vi "DefaultFromIni.vi"(8 "error in (no error)":errorcluster, 11 "CorrFactor in":refnum<class "CorrFactor.lvclass">) -> (0 "error out":errorcluster, 3 "CorrFactor out":refnum<class "CorrFactor.lvclass">)   [LabVIEW 2018, in "AnalysisPlugins.lvlib" / "CorrFactor.lvclass"]
uses:
  CorrFactor.lvclass
  F:/Program Files (x86)/National Instruments/LabVIEW 2018/user.lib/NIST/BaseClasses/BasePlugin_class/BasePlugin.lvclass
  Typedefs/clAnalysisConfig.ctl
  Typedefs/3458 Params.ctl
  <userlib>/NIST/BaseClasses/BasePlugin_class/BasePlugin.lvclass/BasePlugin.ctl
  FGen/MemberClasses/FunctionBaseClass/FunctionBase.lvclass
  CorrFactor.lvclass/CorrFactor.ctl
  <userlib>/NIST/BaseClasses/BasePlugin_class/Accessors/Read PluginIniFilePath.vi
  Accessors/Write 3458_Config.vi
  Accessors/Write FunctionIniFilePath.vi
  Accessors/Write PhaseRange.vi
  Accessors/Write Function.vi
  <vilib>/Utility/error.llb/Error Cluster From Error Code.vi
  FitterBaseClass/FitterBase.lvclass
  <vilib>/ErrorRing/Error Ring.xnode
  <vilib>/Utility/config.llb/NI_LVConfig.lvlib
  <userlib>/NIST/BaseClasses/Object_class/BaseObject.lvclass
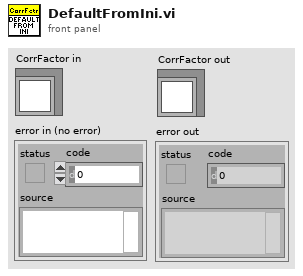
[diagram p1: front panel]
types:
  T1 = typedef "AnalysisPlugins.lvlib/CorrFactor.lvclass/clAnalysisConfig.ctl" = cluster{"HP 3458 address":string, "Amplitude":dbl, "3458  Params:":T2}
  T2 = typedef "AnalysisPlugins.lvlib/CorrFactor.lvclass/3458 Params.ctl" = cluster{"Record Size":i32, "Input Freq (Hz)":dbl, "# Cycles (Desired)":dbl, "Sampling Mode:":u16, "# of Record Avgs./Meas.":i32, "Trigger Mode":u16, "Trig. Level (%)":dbl, "# of Meas. Runs":i32, "Trigger Slope":u16}
  T3 = typedef "NI_LVConfig.lvlib/Config Data RefNum.ctl" = refnum<k1>
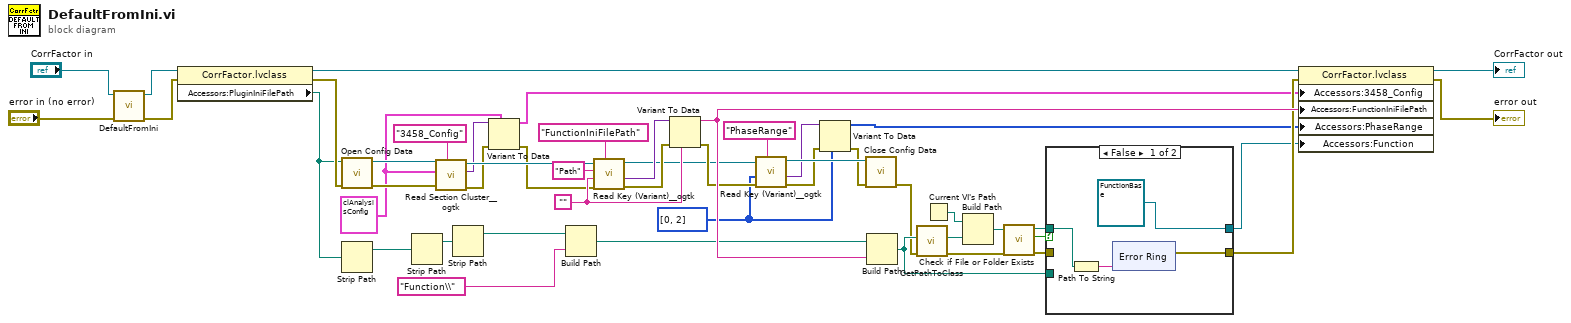
[diagram p0: block diagram]
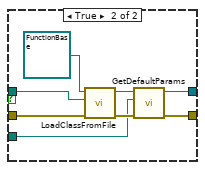
[diagram p2: hidden frame]
diagram:
  w4 = u16[] [0, 2] ("PhaseRange")
  w18 = ""
  w16 = T1 {"HP 3458 address"="", "Amplitude"=0.0, "3458  Params:"={"Record Size"=4096, "Input Freq (Hz)"=50.0, "# Cycles (Desired)"=501.0, "Sampling Mode:"=1, "# of Record Avgs./Meas."=1, "Trigger Mode"=0, "Trig. Level (%)"=0.0, "# of Meas. Runs"=5, "Trigger Slope"=0}} ("clAnalysisConfig")
  n1 = call-parent "DefaultFromIni.vi"("error in (no error)"="error in (no error)", "FitterBase in"="CorrFactor in") -> ("error out"=w45:errorcluster, "FitterBase out"=w49:refnum<class "CorrFactor.lvclass">)  [unwired: 8 in]
  n2 = property class="CorrFactor.lvclass"(reference=w49, error in=w45) -> (reference out=w46:refnum<class "CorrFactor.lvclass">, error out=w44:errorcluster, "Accessors:PluginIniFilePath"=w39:path)
  n3 = call <vilib>:"Open Config Data.vi"("error in (no error)"=w44, "configuration file path"=w39) -> ("error out"=w38:errorcluster, "refnum"=w37:T3)  [unwired: 7 in, 1 out]
  n4 = Strip Path(path=w39) -> (stripped path=w42:path)  [unwired: 1 out]
  n5 = Strip Path(path=w42) -> (stripped path=w41:path)  [unwired: 1 out]
  n6 = call <userlib>:"Read Section Cluster__ogtk.vi"("section (optional)"="3458_Config", "error in (no error)"=w38, "Section Formatted Cluster Type"=w16, "refnum"=w37) -> ("error out"=w14:errorcluster, "Section Formatted Cluster"=w15:variant, "dup refnum"=w35:T3)  [unwired: 3 in, 2 out]
  n7 = Strip Path(path=w41) -> (stripped path=w40:path)  [unwired: 1 out]
  n8 = Variant To Data(error in=w14, type=w16, Variant=w15) -> (data=w12:T1, error out=w13:errorcluster)
  n9 = Build Path(base path=w40, name or relative path="Function\\") -> (appended path=w30:path)
  n10 = call <userlib>:"Read Key (Variant)__ogtk.vi"("section"="FunctionIniFilePath", "error in (no error)"=w13, "type"=w18, "key (optional)"="Path", "refnum"=w35) -> ("error out"=w33:errorcluster, "key-value"=w32:variant, "refnum out"=w7:T3)  [unwired: 3 in, 1 out]
  n11 = Variant To Data(error in=w33, type=w18, Variant=w32) -> (data=w31:string, error out=w8:errorcluster)
  n12 = call <userlib>:"Read Key (Variant)__ogtk.vi"("section"="PhaseRange", "error in (no error)"=w8, "type"=w4, "refnum"=w7) -> ("error out"=w2:errorcluster, "key-value"=w5:variant, "refnum out"=w9:T3)  [unwired: 4 in, 1 out]
  n13 = Variant To Data(error in=w2, type=w4, Variant=w5) -> (data=w3:u16[], error out=w1:errorcluster)
  n14 = call <vilib>:"Close Config Data.vi"("error in (no error)"=w1, "refnum"=w9) -> ("error out"=w28:errorcluster)  [unwired: 8 in, 1 out]
  n15 = Build Path(base path=w30, name or relative path=w31) -> (appended path=w29:path)
  n16 = call <userlib>:"GetPathToClass.vi"("error in (no error)"=w28, "configuration file path"=w29) -> ("error IO"=w25:errorcluster, "PathToClass"=w26:path)  [unwired: 8 in]
  n17 = Current VI's Path() -> (path=w27:path)
  n18 = Build Path(base path=w27, name or relative path=w26) -> (appended path=w24:path)
  n19 = call <vilib>:"Check if File or Folder Exists.vi"("error in (no error)"=w25, "path"=w24) -> ("error out"=w22:errorcluster, "file or folder exists?"=w19:bool, "dup path"=w23:path)  [unwired: 7 in]
  n20 = case shown="False" w19 {
    tunnel: [w52 w63] -> w21
    tunnel: w22 -> [_ w68]
    tunnel: w23 -> [w51 w67]
    tunnel: [refnum<class "FunctionBase.lvclass"> refnum ("Functions.lvlib:FunctionBase.lvclass") w62] -> w10
    tunnel: w29 -> [_ w61]
    frame False {
      n21 = Path To String(path=w51) -> (string=w53:string)
      n22 = xnode "Error Ring"("parameter 0"=w53) -> ("error out"=w52:errorcluster)
    }
    frame True {
      n23 = call-dynamic "LoadClassFromFile.vi"("error in (no error)"=w68, "class path"=w67, "reference in"=refnum<class "FunctionBase.lvclass"> refnum ("Functions.lvlib:FunctionBase.lvclass")) -> ("error out"=w65:errorcluster, "reference out"=w64:refnum<class "FunctionBase.lvclass">)  [unwired: 7 in]
      n24 = call-dynamic "GetDefaultParams.vi"("error in (no error)"=w65, "Path"=w61, "FunctionBase in"=w64) -> ("error out"=w63:errorcluster, "FunctionBase out"=w62:refnum<class "FunctionBase.lvclass">)  [unwired: 7 in]
    }
  }
  n25 = property class="CorrFactor.lvclass"(reference=w46, error in=w21, "Accessors:3458_Config"=w12, "Accessors:FunctionIniFilePath"=w31, "Accessors:PhaseRange"=w3, "Accessors:Function"=w10) -> (reference out=→"CorrFactor out":refnum<class "CorrFactor.lvclass">, error out=→"error out":errorcluster)
